vi "Assemble Archive Headers.vi"(0 "error in":errorcluster) -> (1 "External Sensor Names":string[](array[string]), 2 "error out":errorcluster)   [LabVIEW 2009]
uses:
  Global Data/Names/Name Actions.ctl
  Data Access Objects/Metadata/DAO Actions.ctl
  LogFileType.ctl
  NTCP Client/Control Point Suffix.ctl
  Archive File Type.ctl
panel:
  in  "Command Types":string[](array[string])=["X Cmd Type", "Y Cmd Type", "Z Cmd Type", "RX Cmd Type", "RY Cmd Type", "RZ Cmd Type"]
  in  "Stiffness Column Headers":string[](array[string])=["Column Id", "dFx", "dFy", "dFz", "dMx", "dMy", "dMz"]
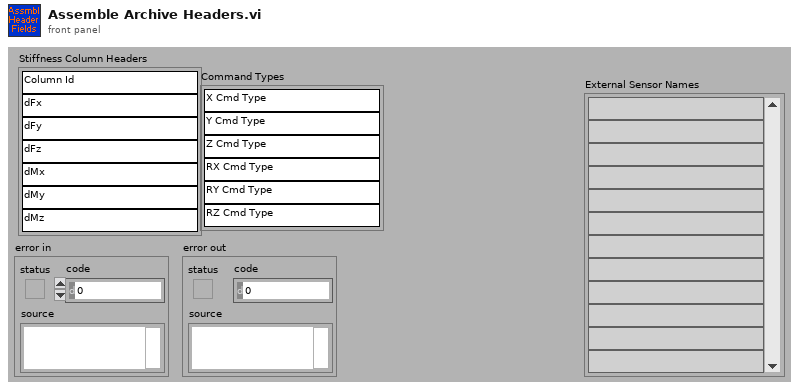
[diagram p1: front panel]
types:
  T1 = typedef "LogFileType.ctl" = enum16{"Continuous", "Step", "Volts", "Offsets", "DLL  Errors", "Snapshot", "Commands", "StiffnessUpdates", "End List"}
  T2 = typedef "Archive File Type.ctl" = enum16{"LBCB1", "LBCB2", "ExternalSensors", "Combined"}
  T3 = typedef "Name Actions.ctl" = enum16{"Init", "Get Names", "Get Index"}
  T4 = typedef "DAO Actions.ctl" = enum16{"Init", "Get", "Set"}
  T5 = typedef "Control Point Suffix.ctl" = enum16{"LBCB1", "LBCB2", "ExternalSensors"}
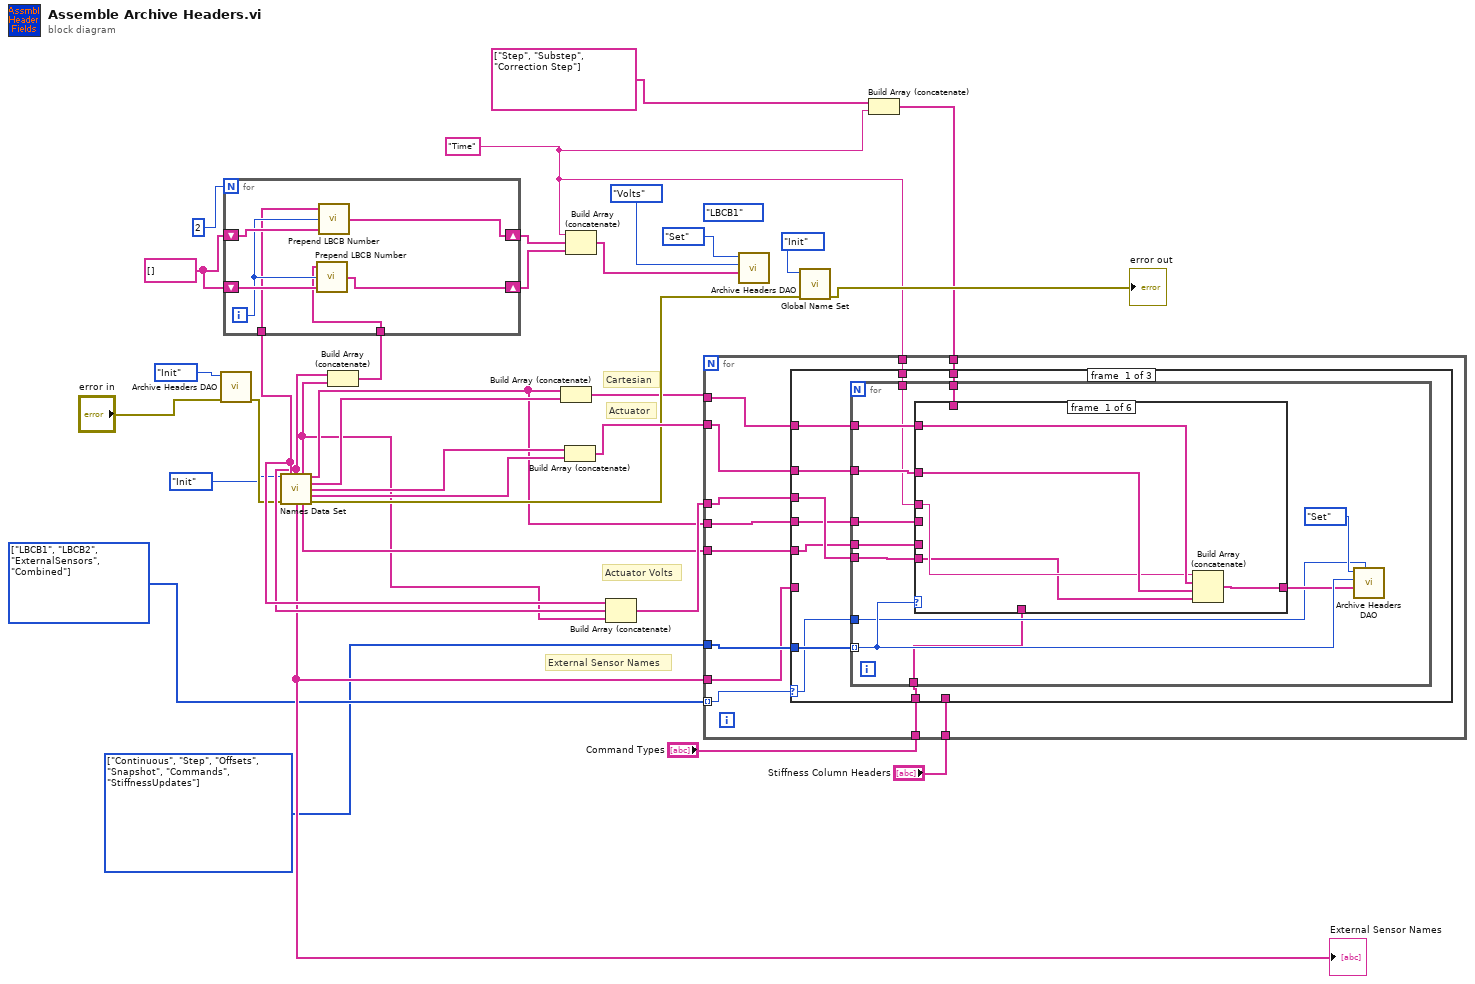
[diagram p0: block diagram]
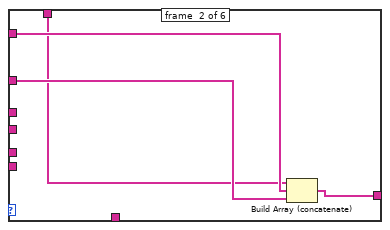
[diagram p2: hidden frame]
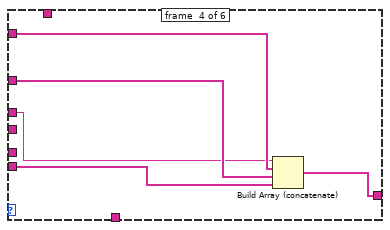
[diagram p4: hidden frame]
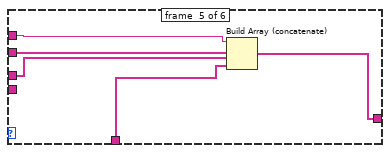
[diagram p5: hidden frame]
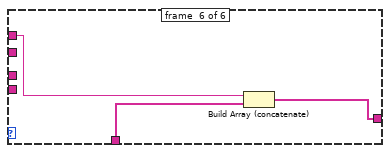
[diagram p6: hidden frame]
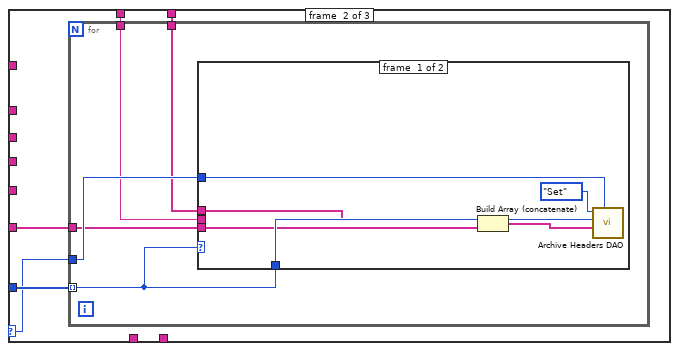
[diagram p7: hidden frame]
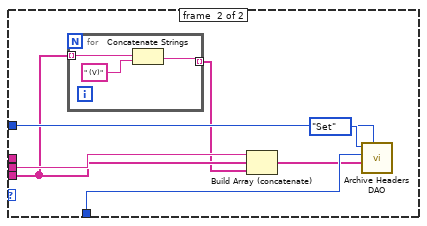
[diagram p8: hidden frame]
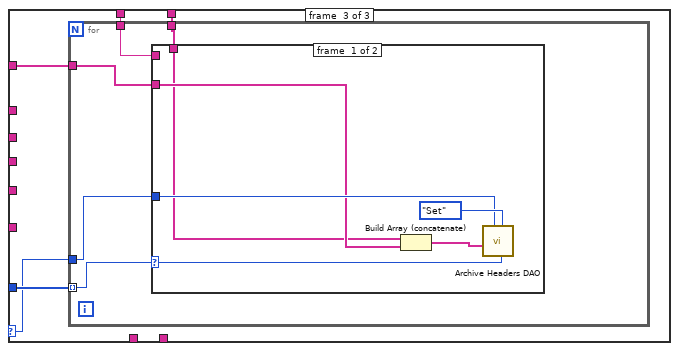
[diagram p9: hidden frame]
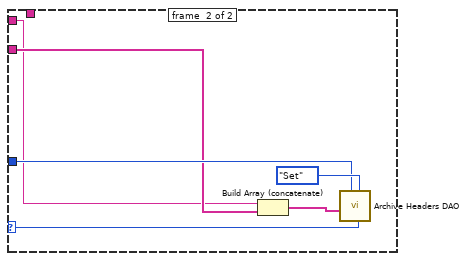
[diagram p10: hidden frame]
diagram:
  w7 = "Time"
  w10 = T1[] [enum."Continuous", enum."Step", enum."Offsets", enum."Snapshot", enum."Commands", enum."StiffnessUpdates"] items=["Continuous", "Step", "Volts", "Offsets", "DLL  Errors", "Snapshot", "Commands", "StiffnessUpdates", "End List"]
  w11 = T2[] [enum."LBCB1", enum."LBCB2", enum."ExternalSensors", enum."Combined"] items=["LBCB1", "LBCB2", "ExternalSensors", "Combined"]
  (unwired) Control_Point_Suffix."LBCB1" ("Contol\nPoint\nSuffix")
  w15 = string[] [] ("Prepended In")
  # "Actuator Volts"
  # "Actuator"
  # "Cartesian"
  # "External Sensor Names"
  n1 = call "Archive Headers DAO.vi"("error in (no error)"="error in", "Actions"=DAO_Actions."Init") -> ("error out"=w25:errorcluster)  [unwired: 3 in, 6 out]
  n2 = call "Names Data Set.vi"("Name Actions"=Name_Actions."Init", "error in (no error)"=w25) -> ("Actuator Command Volts"=w34:string[], "Actuator Volt Readings"=w32:string[], "Servo Names"=w2:string[], "Cartesian Commands"=w5:string[], "Cartesian Readings"=w22:string[], "Actuator Commands"=w17:string[], "Actuator Readings"=w18:string[], "External Sensor Names"=w27:string[], "Cartesian Force Commands"=w4:string[], "error out"=w29:errorcluster)  [unwired: 4 out]
  "External Sensor Names" <- w27
  n3 = Build Array (concatenate)(w32, w2) -> (w9:string[])
  n4 = for {
    N: 2 -> [_]
    tunnel: w34 -> [w36]
    shift-right: [w40] -> w14
    shift-left: w15 -> [w41]
    shift-right: [w38] -> w16
    shift-left: w15 -> [w39]
    tunnel: w9 -> [w35]
    i -> [w37]
    n5 = call "Prepend LBCB Number.vi"("Prepended In"=w41, "LBCB Number"=w37, "Names In"=w35) -> ("Prepended Out"=w40:string[])
    n6 = call "Prepend LBCB Number.vi"("Prepended In"=w39, "LBCB Number"=w37, "Names In"=w36) -> ("Prepended Out"=w38:string[])
  }
  n7 = Build Array (concatenate)(w5, w22) -> (w23:string[])
  n8 = Build Array (concatenate)(w17, w18) -> (w31:string[])
  n9 = Build Array (concatenate)(w7, w16, w14) -> (w20:string[])
  n10 = Build Array (concatenate)(w34, w32, w2) -> (w33:string[])
  n11 = call "Archive Headers DAO.vi"("Headers In"=w20, "LogFile Type"=LogFileType."Volts", "Actions"=DAO_Actions."Set") -> ()  [unwired: 2 in, 7 out]
  n12 = call "Global Name Set.vi"("error in (no error)"=w29, "Name Actions"=Name_Actions."Init") -> ("error out"=→"error out":errorcluster)  [unwired: 1 in, 8 out]
  n13 = Build Array (concatenate)(string[] ["Step", "Substep", "Correction Step"], w7) -> (w6:string[])
  n14 = for {
    tunnel: w23 -> [w52]
    tunnel: w27 -> [w48]
    tunnel: w31 -> [w51]
    tunnel: w33 -> [w50]
    tunnel: w11 -> [w49] mode=indexing
    tunnel: w10 -> [w53]
    tunnel: w7 -> [w47]
    tunnel: w6 -> [w46]
    tunnel: w5 -> [w45]
    tunnel: w4 -> [w44]
    tunnel: "Stiffness Column Headers" -> [w43]
    tunnel: "Command Types" -> [w42]
    n15 = case shown="\"LBCB1\", Default" w49 {
      selector: w49 -> [w57 w99 w125]
      tunnel: w53 -> [w63 w103 w129]
      tunnel: w52 -> [w62 _ w128]
      tunnel: w51 -> [w61 _ _]
      tunnel: w50 -> [w60 _ _]
      tunnel: w48 -> [_ w102 _]
      tunnel: w47 -> [w59 w101 w127]
      tunnel: w46 -> [w58 w100 w126]
      tunnel: w45 -> [w55 _ _]
      tunnel: w44 -> [w54 _ _]
      tunnel: w43 -> [_ _ _]
      tunnel: w42 -> [w56 _ _]
      frame #0 {
        n16 = for {
          tunnel: w63 -> [w74] mode=indexing
          tunnel: w62 -> [w73]
          tunnel: w61 -> [w72]
          tunnel: w60 -> [w70]
          tunnel: w57 -> [w69]
          tunnel: w59 -> [w68]
          tunnel: w58 -> [w67]
          tunnel: w56 -> [w66]
          tunnel: w55 -> [w65]
          tunnel: w54 -> [w64]
          n17 = case shown="\"StiffnessUpdates\"" w74 {
            tunnel: w73 -> [w80 w84 w85 w90 _ _]
            tunnel: w72 -> [w79 w83 _ w89 _ _]
            tunnel: [w78 w82 w85 w87 w92 w96] -> w71
            tunnel: w70 -> [w76 _ _ w88 _ _]
            tunnel: w68 -> [w77 _ _ w86 w91 w98]
            tunnel: w67 -> [_ w81 _ _ _ _]
            tunnel: w66 -> [_ _ _ _ w95 w97]
            tunnel: w65 -> [_ _ _ _ w94 _]
            tunnel: w64 -> [_ _ _ _ w93 _]
            frame #0 {
              n18 = Build Array (concatenate)(w77, w80, w79, w76) -> (w78:string[])
            }
            frame #1 {
              n19 = Build Array (concatenate)(w81, w84, w83) -> (w82:string[])
            }
            frame #2 {
            }
            frame #3 {
              n20 = Build Array (concatenate)(w86, w90, w89, w88) -> (w87:string[])
            }
            frame #4 {
              n21 = Build Array (concatenate)(w91, w94, w93, w95) -> (w92:string[])
            }
            frame #5 {
              n22 = Build Array (concatenate)(w98, w97) -> (w96:string[])
            }
          }
          n23 = call "Archive Headers DAO.vi"("Archive File Type"=w69, "Headers In"=w71, "LogFile Type"=w74, "Actions"=DAO_Actions."Set") -> ()  [unwired: 1 in, 7 out]
        }
      }
      frame #1 {
        n24 = for {
          tunnel: w103 -> [w105] mode=indexing
          tunnel: w99 -> [w108]
          tunnel: w102 -> [w107]
          tunnel: w101 -> [w106]
          tunnel: w100 -> [w104]
          n25 = case shown="\"Continuous\", Default" w105 {
            tunnel: w105 -> [w113 w120]
            tunnel: w108 -> [w112 w119]
            tunnel: w107 -> [w111 w116]
            tunnel: w106 -> [_ w117]
            tunnel: w104 -> [w109 _]
            frame #0 {
              n26 = Build Array (concatenate)(w109, w111) -> (w110:string[])
              n27 = call "Archive Headers DAO.vi"("Archive File Type"=w112, "Headers In"=w110, "LogFile Type"=w113, "Actions"=DAO_Actions."Set") -> ()  [unwired: 1 in, 7 out]
            }
            frame #1 {
              n28 = for {
                tunnel: w116 -> [w124] mode=indexing
                tunnel: [w122] -> w115 mode=indexing
                n29 = Concatenate Strings(w124, " (V)" ("string")) -> (w122:string)
              }
              n30 = Build Array (concatenate)(w117, w116, w115) -> (w118:string[])
              n31 = call "Archive Headers DAO.vi"("Archive File Type"=w119, "Headers In"=w118, "LogFile Type"=w120, "Actions"=DAO_Actions."Set") -> ()  [unwired: 1 in, 7 out]
            }
          }
        }
      }
      frame #2 {
        n32 = for {
          tunnel: w129 -> [w131] mode=indexing
          tunnel: w128 -> [w133]
          tunnel: w125 -> [w134]
          tunnel: w127 -> [w132]
          tunnel: w126 -> [w130]
          n33 = case shown="\"Volts\", Default" w131 {
            selector: w131 -> [w136 w142]
            tunnel: w134 -> [w139 w145]
            tunnel: w133 -> [w138 w144]
            tunnel: w132 -> [_ w141]
            tunnel: w130 -> [w135 _]
            frame #0 {
              n34 = Build Array (concatenate)(w135, w138) -> (w137:string[])
              n35 = call "Archive Headers DAO.vi"("Archive File Type"=w139, "Headers In"=w137, "LogFile Type"=w136, "Actions"=DAO_Actions."Set") -> ()  [unwired: 1 in, 7 out]
            }
            frame #1 {
              n36 = Build Array (concatenate)(w141, w144) -> (w143:string[])
              n37 = call "Archive Headers DAO.vi"("Archive File Type"=w145, "Headers In"=w143, "LogFile Type"=w142, "Actions"=DAO_Actions."Set") -> ()  [unwired: 1 in, 7 out]
            }
          }
        }
      }
    }
  }
